vi "Write Light Select.vi"(8 "error in (no error)":errorcluster, 10 "Light Select":T1, 11 "Light Stack in":refnum<class "Light Stack.lvclass">) -> (0 "error out":errorcluster, 3 "Light Stack out":refnum<class "Light Stack.lvclass">)   [LabVIEW 2018, in "Light Stack.lvlib" / "Light Stack.lvclass"]
uses:
  Light Stack.lvclass
  Custom Controls/Light Select.ctl
  Light Stack.lvclass/Light Stack.ctl
  Light Stack.lvlib
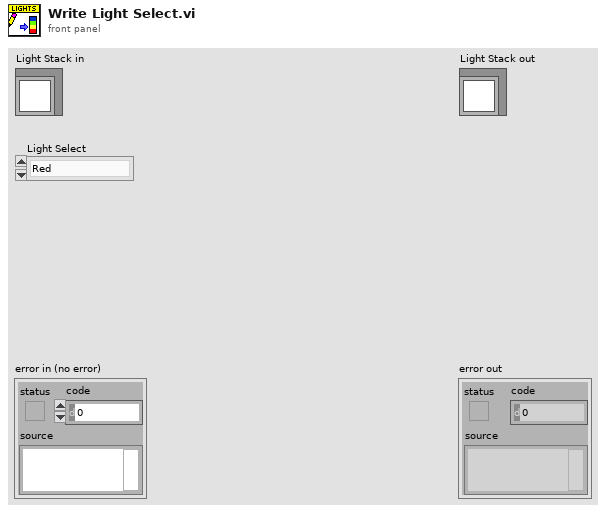
[diagram p1: front panel]
types:
  T1 = typedef "Light Stack.lvlib/Light Select.ctl" = enum16{"Red", "Amber", "Green", "Blue"}
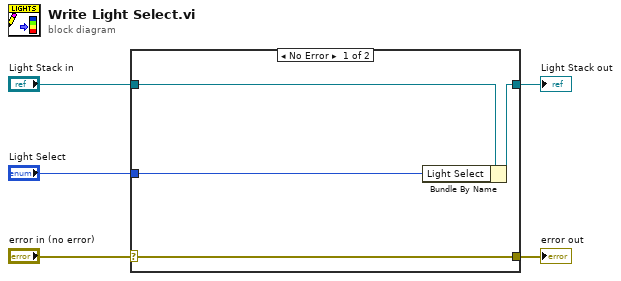
[diagram p0: block diagram]
diagram:
  n1 = case shown="No Error" "error in (no error)" {
    selector: "error in (no error)" -> [w9 w10]
    tunnel: [w9 w10] -> w4
    tunnel: [w7 w11] -> w2
    tunnel: "Light Stack in" -> [w8 w11]
    tunnel: "Light Select" -> [w6 _]
    frame No Error {
      n2 = Bundle By Name(cluster=w8, "Light Select"=w6) -> (w7:refnum<class "Light Stack.lvclass">)
    }
    frame Error {
    }
  }
  "error out" <- w4
  "Light Stack out" <- w2
